vi "GetConfig.vi"(8 "error in (no error)":errorcluster) -> (0 "error out":errorcluster, 3 "Config":T1={"Path"="C:\\Glass", "Days to Keep"=30, "Number of Rows"=90})   [LabVIEW 2015, in "ConfigHelper.lvlib"]
uses:
  ConfigHelper.lvlib
  Config.ctl
  <vilib>/addons/PointValueMap/subVIs/Point_Read_variant.vi
  <vilib>/addons/PointValueMap/PointValueMap.lvlib
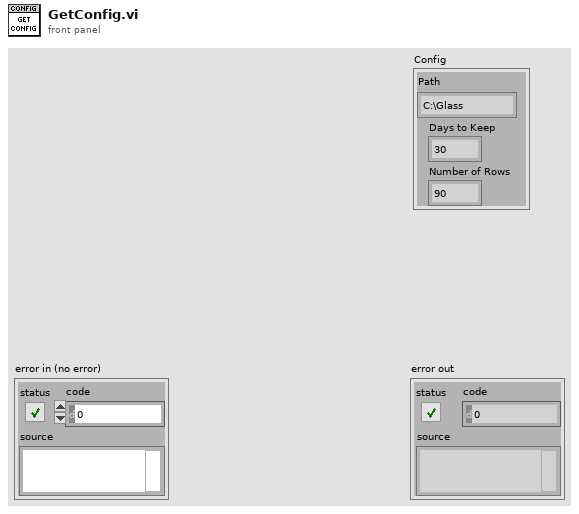
[diagram p1: front panel]
types:
  T1 = typedef "ConfigHelper.lvlib/Config.ctl" = cluster{"Path":string, "Days to Keep":i32, "Number of Rows":i32}
  T2 = typedef "PointValueMap.lvlib/PointMap.ctl" = refnum<data-value>
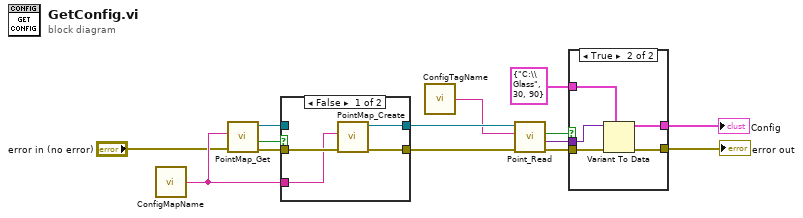
[diagram p0: block diagram]
diagram:
  n1 = call "ConfigMapName.vi"() -> ("Name"=w9:string)  [unwired: 5 in]
  n2 = call <vilib>:"PointMap_Get.vi"("error in (no error)"="error in (no error)", "Name"=w9) -> ("error out"=w13:errorcluster, "Found?"=w14:bool, "Map Out"=w12:T2)  [unwired: 7 in]
  n3 = case shown="False" w14 {
    tunnel: w13 -> [w18 w19]
    tunnel: w12 -> [_ w20]
    tunnel: w9 -> [w17 _]
    tunnel: [w16 w20] -> w10
    tunnel: [w15 w19] -> w11
    frame False {
      n4 = call <vilib>:"PointMap_Create.vi"("error in (no error)"=w18, "Name"=w17) -> ("error out"=w15:errorcluster, "Map Out"=w16:T2)  [unwired: 8 in]
    }
    frame True {
    }
  }
  n5 = call "ConfigTagName.vi"() -> ("Name"=w8:string)  [unwired: 5 in]
  n6 = call-poly <vilib>:"Point_Read.vi"("Error In"=w11, "Tag"=w8, "Map"=w10) -> ("Error Out"=w6:errorcluster, "Value"=w4:variant, "Found?"=w5:bool)  [unwired: 3 in, 3 out]
  n7 = case shown="True" w5 {
    tunnel: w6 -> [w21 w27]
    tunnel: w4 -> [_ w26]
    tunnel: T1 {"Path"="C:\\Glass", "Days to Keep"=30, "Number of Rows"=90} ("Config") -> [w22 w25]
    tunnel: [w22 w24] -> w1
    tunnel: [w21 w23] -> w2
    frame False {
    }
    frame True {
      n8 = Variant To Data(error in=w27, type=w25, Variant=w26) -> (data=w24:T1, error out=w23:errorcluster)
    }
  }
  "error out" <- w2
  "Config" <- w1
